vi "1. MassData Argument Format.vi"() -> ()   [LabVIEW 2017]
doc: "## MassData Argument Format (1. MassData Argument Format.vi)\n\n### Overview\n\nMassData arguments are used within the CSM framework to transfer large amounts of data, such as arrays and waveform data. MassData arguments are also used for lossless transfer of complex data types. This example demonstrates the MassData argument formats supported by the CSM API.\n\n### Introduction\n\nThis example simulates the generation of two sets of data: a set of I32 array data and a set of waveform data. Both sets are converted into MassData arguments.\n\nCSM supports the following MassData argument format:\n\n```\n<massdata>Start:8057;Size:4004;DataType:1D I32\n```\n\nThe meaning of each part is as follows:\n\n- `<massdata>`: Indicates that this is a MassData argument.\n- `Start`: The starting address of the MassData in memory.\n- `Size`: The size of the MassData (in bytes).\n- `DataType`: (Optional) The data type of the MassData. Depending on the conversion function selected, this part may not be included.\n\n### Steps\n\n- Step 1: I32 array data. The conversion function selected for this step is `CSM - Convert MassData to Argument With DataType.vim`, so it includes the `DataType` section.\n - Step 1.1: Construct raw data, which in a real-world program comes from hardware acquisition, data reception, etc.\n - Step 1.2: Call `CSM - Convert MassData to Argument With DataType.vim` to convert the raw data into a MassData argument. You can view the converted argument format on the front panel.\n - Step 1.3: Use `CSM - MassData Data Type String.vi` to retrieve the data type from the MassData argument string.\n - Step 1.4: Use `CSM - Argument Type.vi` to retrieve the CSM argument tag, which in this case is `<massdata>`.\n - Step 1.5: Convert the MassData argument back to raw data. You can view the converted data on the front panel. The converted data should match the original data exactly.\n- Step 2: Waveform Data. The conversion function selected for this section is `CSM - Convert MassData to Argument.vim`, so it does not include the `DataType` section.\n - Step 2.1: Construct raw data, which in a real-world program comes from hardware acquisition, data reception, etc.\n - Step 2.2: Call `CSM - Convert MassData to Argument.vim` to convert the raw data into a MassData argument. You can view the converted argument format on the front panel. The `DataType` section is not included.\n - Step 2.3: Use `CSM - Argument Type.vi` to retrieve the CSM argument tag, which in this case is `<massdata>`.\n - Step 2.4: Convert the MassData argument back to raw data. You can view the converted data on the front panel. The converted data should match the original data exactly."
uses:
  d9b05c6c-ba81-4115-93d2-667856f49ac3.vi
  d3df8c6a-f03e-4c4e-bd98-6e1e31b82a4e.vi
  71debf07-57be-4e84-83e8-2003debbe77f.vi
  97537ff4-639f-415a-91df-e0656b80dba4.vi
  <userlib>/_NEVSTOP/Communicable State Machine(CSM)/Utility/CSM Data Type String.vi
  addons/MassData-Parameter/_support/FGV-MassData(lvlibp).vi
  <userlib>/_NEVSTOP/Communicable State Machine(CSM)/_Shared/CSM Shared.lvlib
  addons/MassData-Parameter/CSM MassData Parameter Support.lvlib
panel:
  out "Data Type String 1":string
  out "CSM Argument(as <massdata>) 2":string
  out "Arg Token 2":string
  out "Arg Token 1":string
  out "unpacked source data 2":waveform(dbl)(graph)
  out "unpacked source data 1":i32[](graph)
  out "CSM Argument(as <massdata>) 1":string
  # "#CSM-Example overview\n\nMassData arguments are used within the CSM framework to transfer large amounts of data, such as arrays and waveform data. MassData arguments are also used for lossless transfer of complex data types. This example demonstrates the MassData argument formats supported by the CSM API."
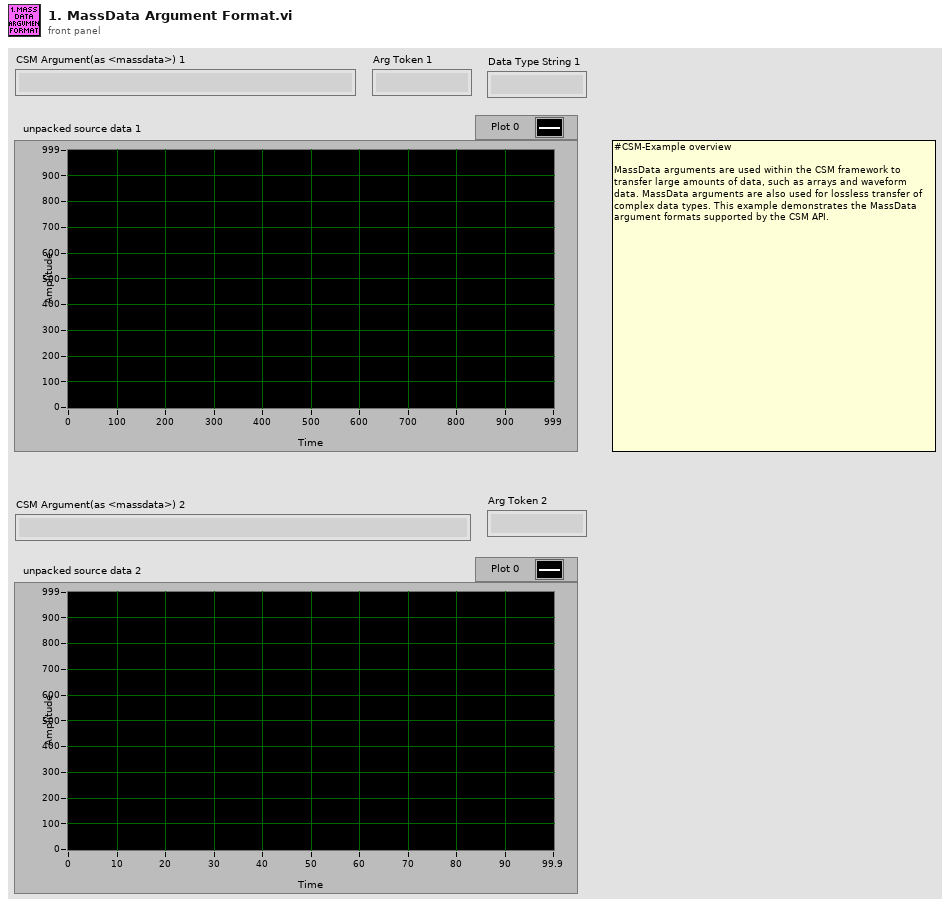
[diagram p1: front panel]
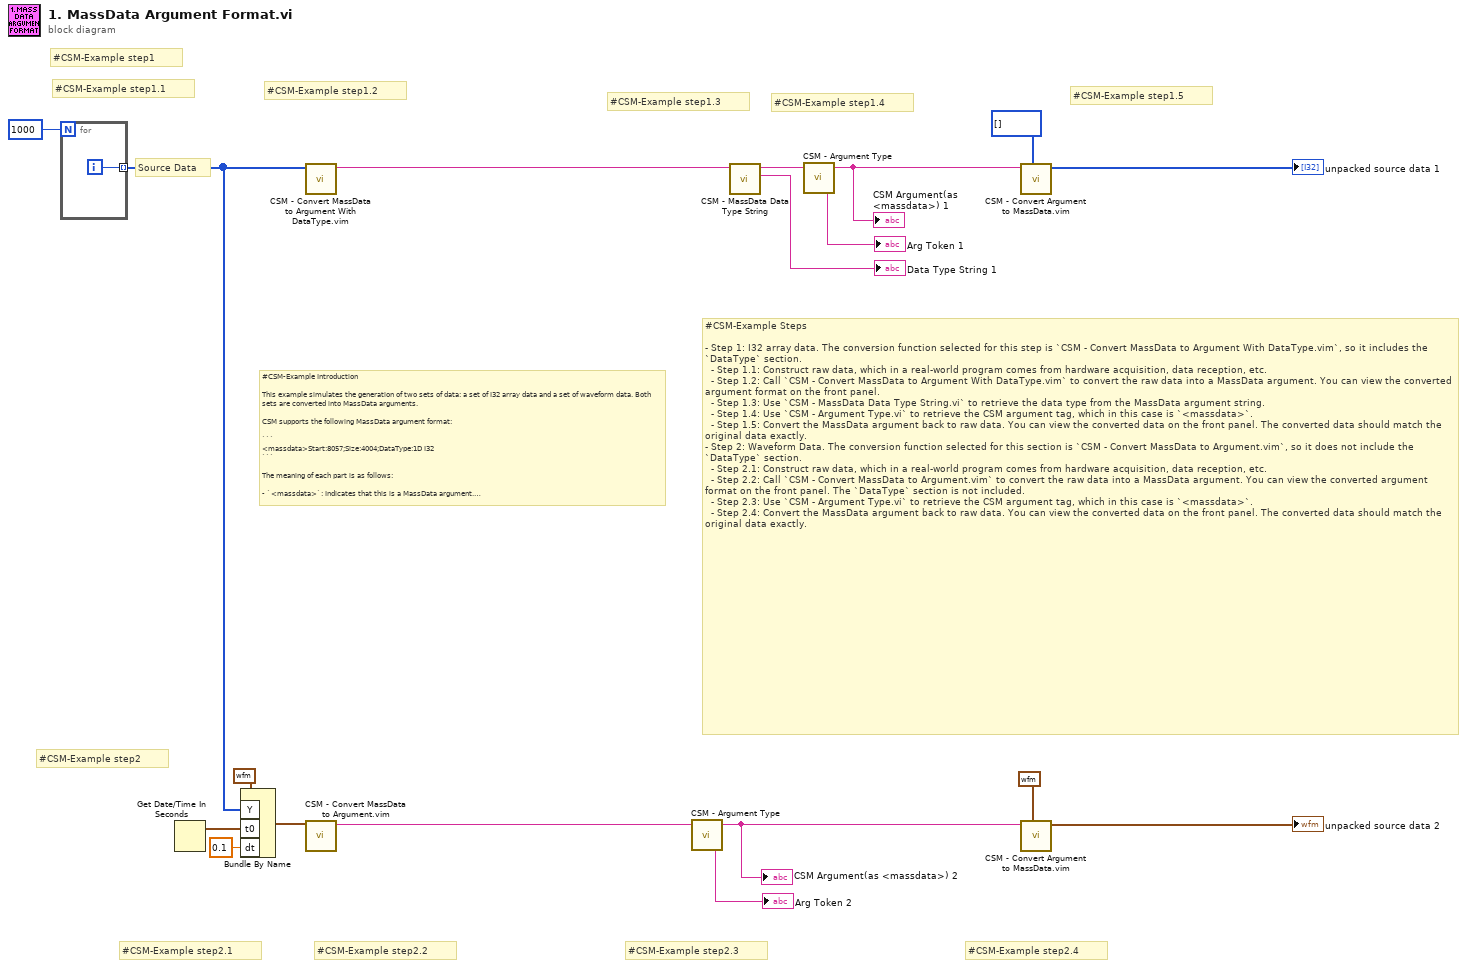
[diagram p0: block diagram]
diagram:
  # "#CSM-Example step1.5"
  # "#CSM-Example step1.4"
  # "#CSM-Example step1.3"
  # "#CSM-Example step1.2"
  # "#CSM-Example step2.4"
  # "#CSM-Example step2.3"
  # "#CSM-Example step2.2"
  # "#CSM-Example step2.1"
  # "#CSM-Example step1.1"
  # "#CSM-Example step2"
  # "#CSM-Example step1"
  # "#CSM-Example Steps\n\n- Step 1: I32 array data. The conversion function selected for this step is `CSM - Convert MassData to Argument With DataType.vim`, so it includes the `DataType` section.\n  - Step 1.1: Construct raw data, which in a real-world program comes from hardware acquisition, data reception, etc.\n  - Step 1.2: Call `CSM - Convert MassData to Argument With DataType.vim` to convert the raw data into a MassData argument. You can view the converted argument format on the front panel.\n  - Step 1.3: Use `CSM - MassData Data Type String.vi` to retrieve the data type from the MassData argument string.\n  - Step 1.4: Use `CSM - Argument Type.vi` to retrieve the CSM argument tag, which in this case is `<massdata>`.\n  - Step 1.5: Convert the MassData argument back to raw data. You can view the converted data on the front panel. The converted data should match the original data exactly.\n- Step 2: Waveform Data. The conversion function selected for this section is `CSM - Convert MassData to Argument.vim`, so it does not include the `DataType` section.\n  - Step 2.1: Construct raw data, which in a real-world program comes from hardware acquisition, data reception, etc.\n  - Step 2.2: Call `CSM - Convert MassData to Argument.vim` to convert the raw data into a MassData argument. You can view the converted argument format on the front panel. The `DataType` section is not included.\n  - Step 2.3: Use `CSM - Argument Type.vi` to retrieve the CSM argument tag, which in this case is `<massdata>`.\n  - Step 2.4: Convert the MassData argument back to raw data. You can view the converted data on the front panel. The converted data should match the original data exactly."
  # "#CSM-Example Introduction\n\nThis example simulates the generation of two sets of data: a set of I32 array data and a set of waveform data. Both sets are converted into MassData arguments.\n\nCSM supports the following MassData argument format:\n\n```\n<massdata>Start:8057;Size:4004;DataType:1D I32\n```\n\nThe meaning of each part is as follows:\n\n- `<massdata>`: Indicates that this is a MassData argument.\n- `Start`: The starting address of the MassData in memory.\n- `Size`: The size of the MassData (in bytes).\n- `DataType`: (Optional) The data type of the MassData. Depending on the conversion function selected, this part may not be included."
  # "Source Data"
  n1 = for {
    N: 1000 -> [_]
    tunnel: [w19] -> w5 mode=indexing
    i -> [w19]
  }
  n2 = Get Date/Time In Seconds() -> (seconds since 1Jan1904=w8:timestamp)
  n3 = Bundle By Name(cluster=waveform(dbl) {"t0"=timestamp(0 s since 1904-01-01), "dt"=1.0, "Y"=[]} ("Waveform"), "Y"=w5, "t0"=w8, "dt"=0.1) -> (w4:waveform(dbl))
  n4 = call "CSM - Convert MassData to Argument With DataType.vim"("Data"=w5) -> ("MassData Argument"=w3:string)  [unwired: 7 in, 1 out]
  n5 = call "CSM - Convert MassData to Argument.vim"("Data"=w4) -> ("MassData Argument"=w11:string)  [unwired: 7 in, 1 out]
  n6 = call <userlib>:"CSM - Argument Type.vi"("Arguments"=w11) -> ("Argument Type"=→"Arg Token 2":string, "Arguments (Dup)"=w10:string)  [unwired: 3 in]
  "CSM Argument(as <massdata>) 2" <- w10
  n7 = call "CSM - MassData Data Type String.vi"("MassData Argument"=w3) -> ("Data Type String"=→"Data Type String 1":string, "MassData Argument (dup)"=w2:string)  [unwired: 6 in, 1 out]
  n8 = call <userlib>:"CSM - Argument Type.vi"("Arguments"=w2) -> ("Argument Type"=→"Arg Token 1":string, "Arguments (Dup)"=w13:string)  [unwired: 3 in]
  "CSM Argument(as <massdata>) 1" <- w13
  n9 = call "CSM - Convert Argument to MassData.vim"("Type"=i32[] [], "MassData Argument"=w13) -> ("Data"=→"unpacked source data 1":i32[])  [unwired: 6 in, 1 out]
  n10 = call "CSM - Convert Argument to MassData.vim"("Type"=waveform(dbl) {"t0"=timestamp(0 s since 1904-01-01), "dt"=1.0, "Y"=[]} ("Waveform"), "MassData Argument"=w10) -> ("Data"=→"unpacked source data 2":waveform(dbl))  [unwired: 6 in, 1 out]
